vi "Feed Manager.vi"() -> ()   [LabVIEW 2014]
uses:
  _support/Feed Manager States.ctl
  _support/Feed Manager State Data.ctl
  _support/Feed Info.ctl
  _support/UI references.ctl
  <vilib>/Utility/miscctls.llb/LVRowAndColumnTypeDef.ctl
  <vilib>/Utility/miscctls.llb/LVRowAndColumnUnsignedTypeDef.ctl
  <vilib>/National Instruments/NIPM API (Beta)/NIPM_API.lvlib
panel:
  in  "Help Button":bool
  out "Package Attributes":string[][](table)
  in  "Refresh":bool
  in  "Packages in Feed":i32(listbox)=-1
  in  "Unpublish Package":bool
  in  "Publish Package":bool
  in  "Configure Feeds":bool
  in  "Feed":string(combo)="Select a Feed..."
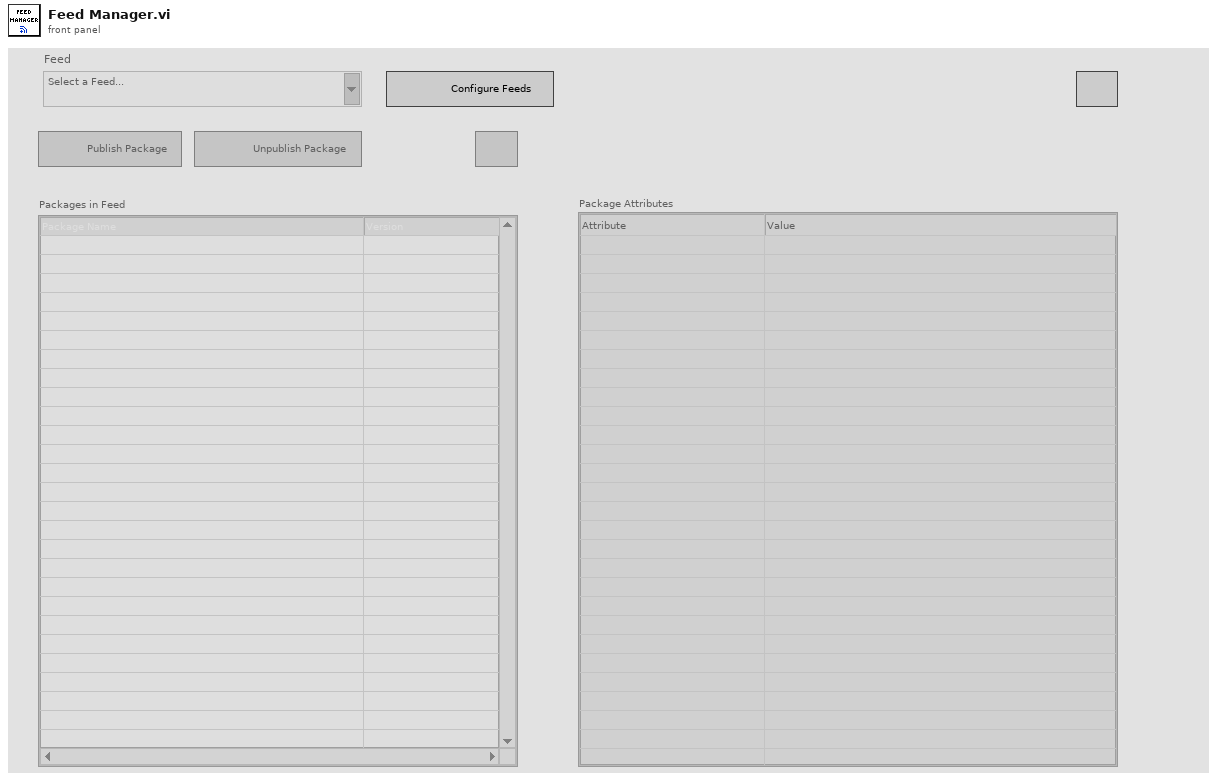
[diagram p1: front panel]
types:
  T1 = typedef "Feed Manager State Data.ctl" = cluster{"Feeds INI Filepath":path, "Current Feed":T2, "Current Row Index":i32, "Managed Feeds":T2[], "Temp Registered Feeds":T2[], "Temp Feed Prefix":string, "Package Relative Filepaths":path[], "UI References":T3}
  T2 = typedef "Feed Info.ctl" = cluster{"Feed Name":string, "Feed Folderpath":string, "Package Destination Folderpath":string}
  T3 = typedef "UI references.ctl" = cluster{"Publish Package":refnum<vi>, "Unpublish Package":refnum<vi>, "Refresh":refnum<vi>, "Packages in Feed":refnum<vi>, "Package Attributes":refnum<vi>}
  T4 = typedef "Feed Manager States.ctl" = enum16{"Initialize", "Wait on Event", "Update Available Feeds", "Configure Feeds", "Update Packages Table", "Update Package Attributes Display", "Publish Package", "Unpublish Package", "Refresh Feed", "Exit"}
  T5 = typedef "LVRowAndColumnTypeDef.ctl" = cluster{"Row":i32, "Column":i32}
  T6 = enum8{"Enabled", "Disabled", "Disabled and Grayed Out"}
  T7 = typedef "LVRowAndColumnUnsignedTypeDef.ctl" = cluster{"Row":u32, "Column":u32}
  T8 = typedef "NIPM_API.lvlib/feed.ctl" = cluster{"Name":string, "URI":string}
  T9 = typedef "NIPM_API.lvlib/package attributes.ctl" = cluster{"Package Name":string, "Display name":string, "Version":string, "Display version":string, "Synopsis":string, "Description":string, "Maintainer":string, "Maintainer email address":string, "Category":string, "Homepage":string, "Release notes":string, "Depends":string[], "Recommends":string[], "Suggests":string[], "Conflicts":string[], "Provides":string[], "Replaces":string[], "Supplements":string[], "Enhances":string[], "Product":bool, "User visible":bool, "Installed size (KB)":u64, "Package filesize (bytes)":u64, "Architecture":string, "Agent":string, "MD5Checksum":string}
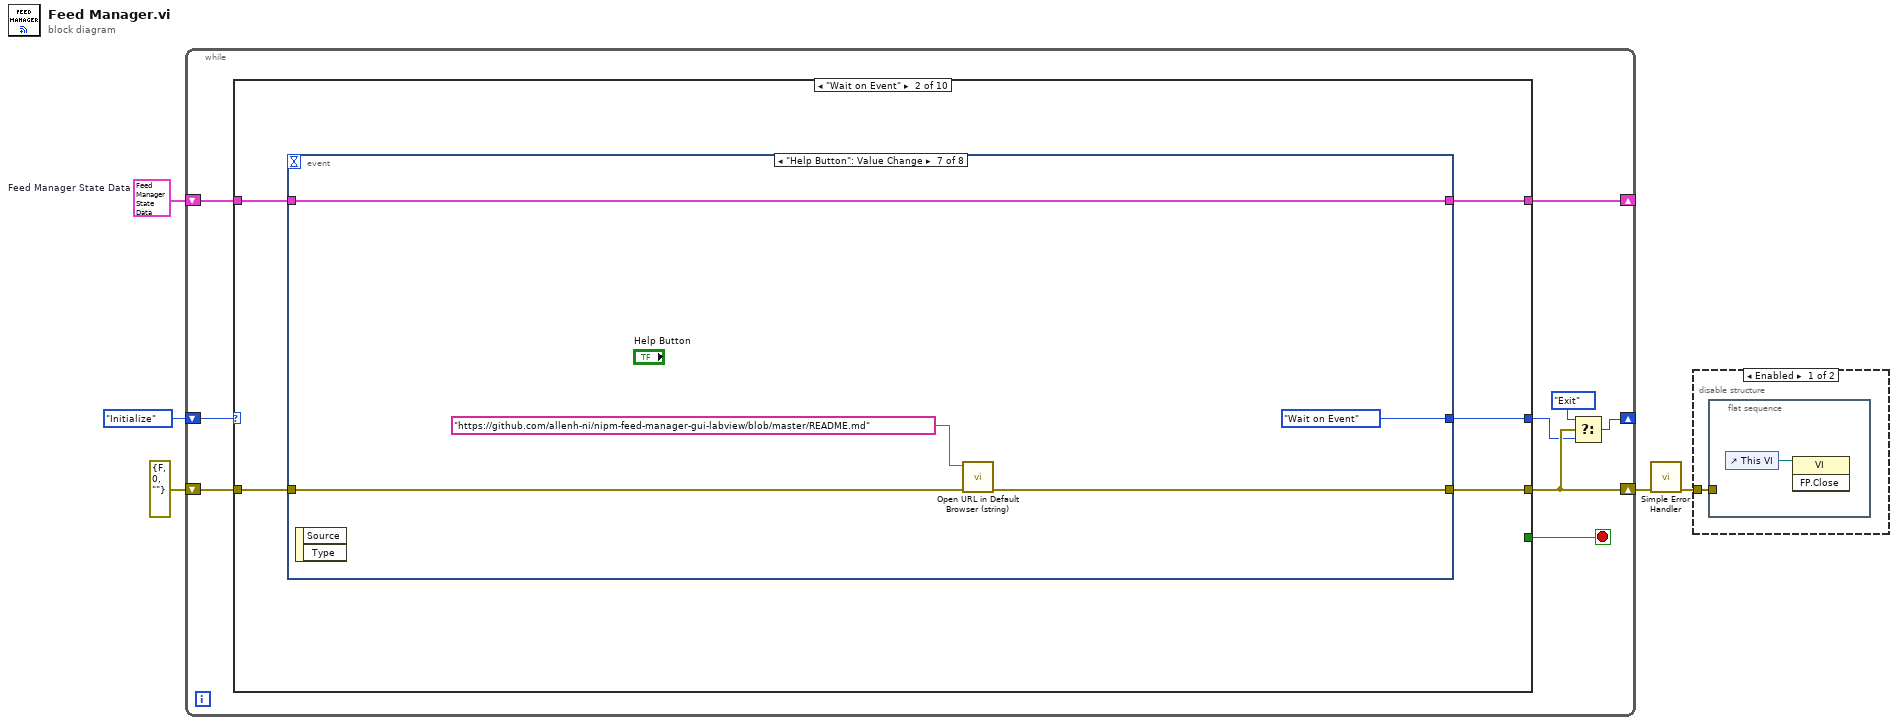
[diagram p0: block diagram]
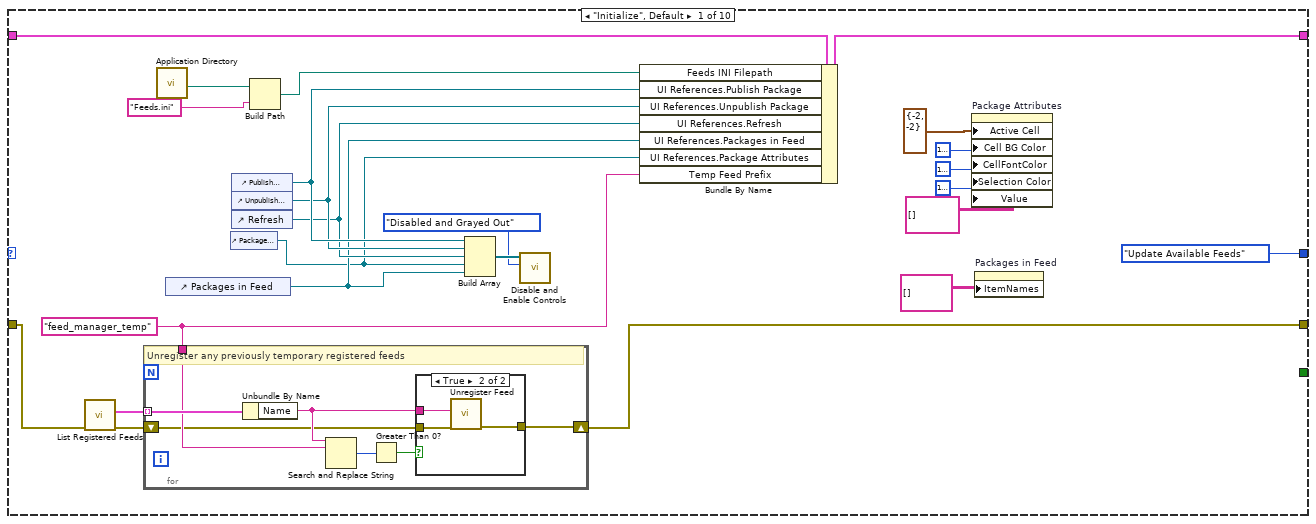
[diagram p3: hidden frame]
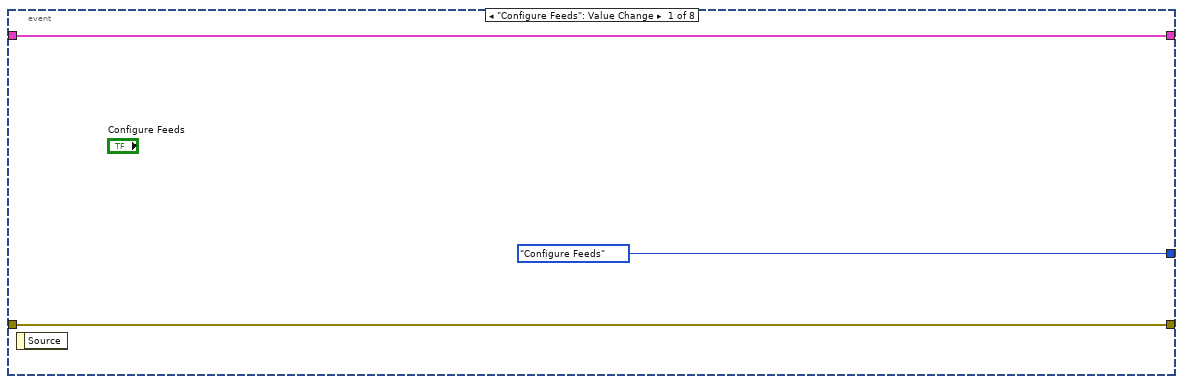
[diagram p5: hidden frame]
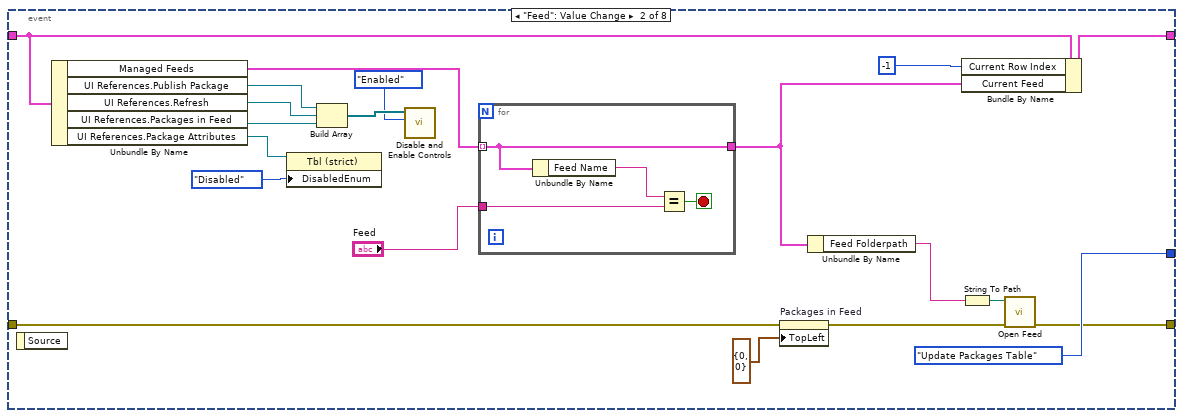
[diagram p6: hidden frame]
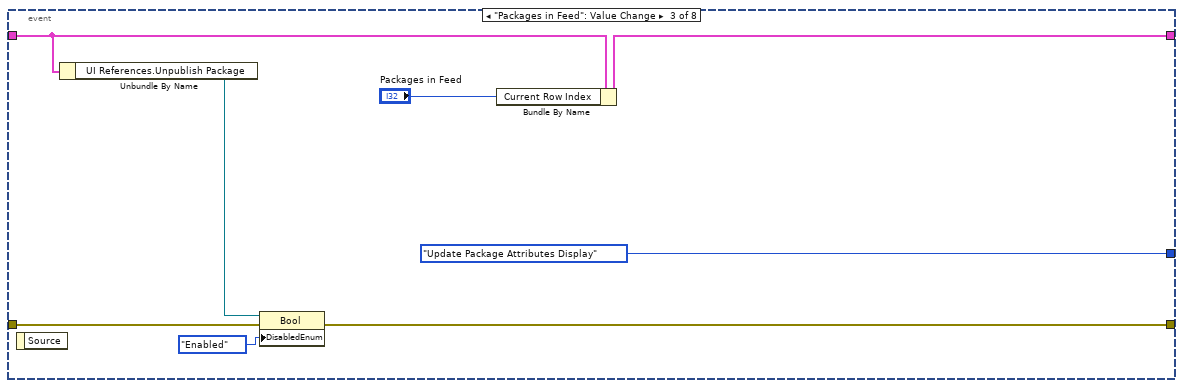
[diagram p7: hidden frame]
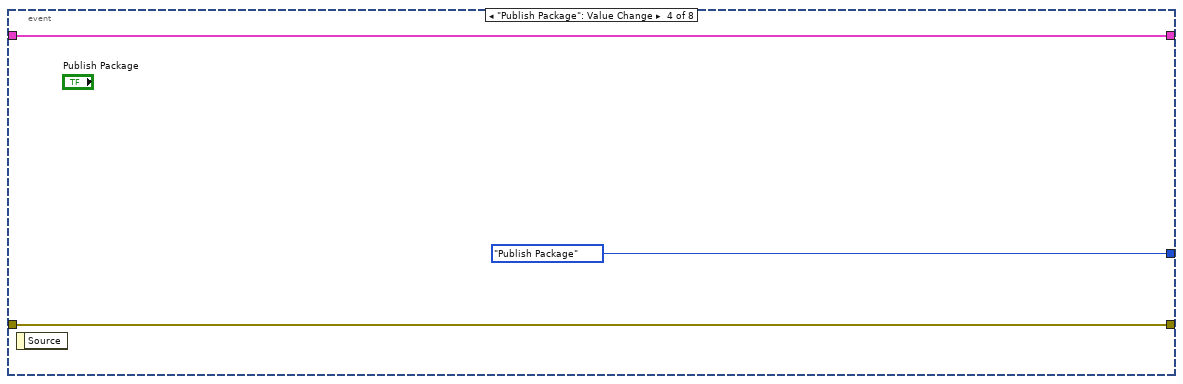
[diagram p8: hidden frame]
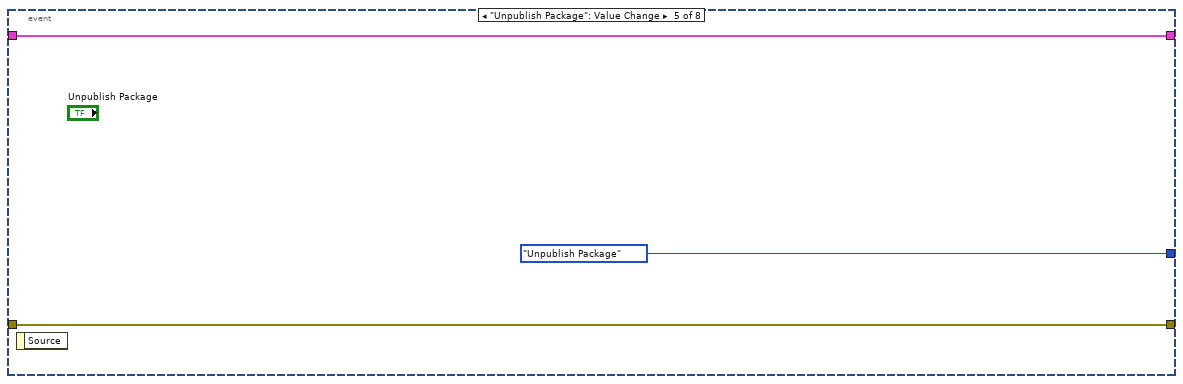
[diagram p9: hidden frame]
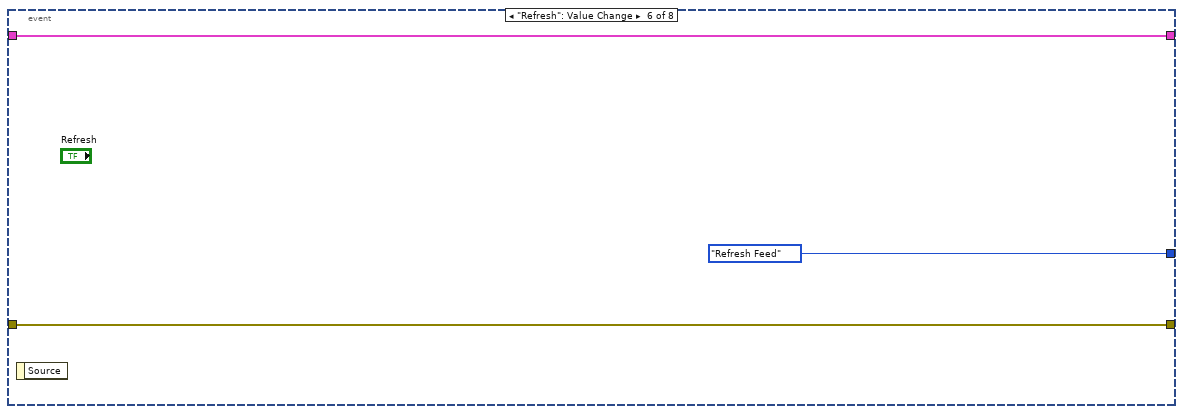
[diagram p10: hidden frame]
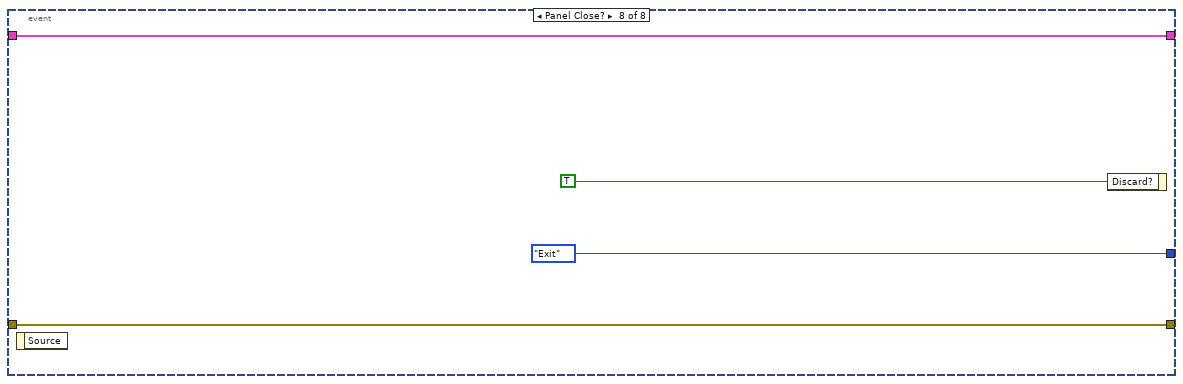
[diagram p11: hidden frame]
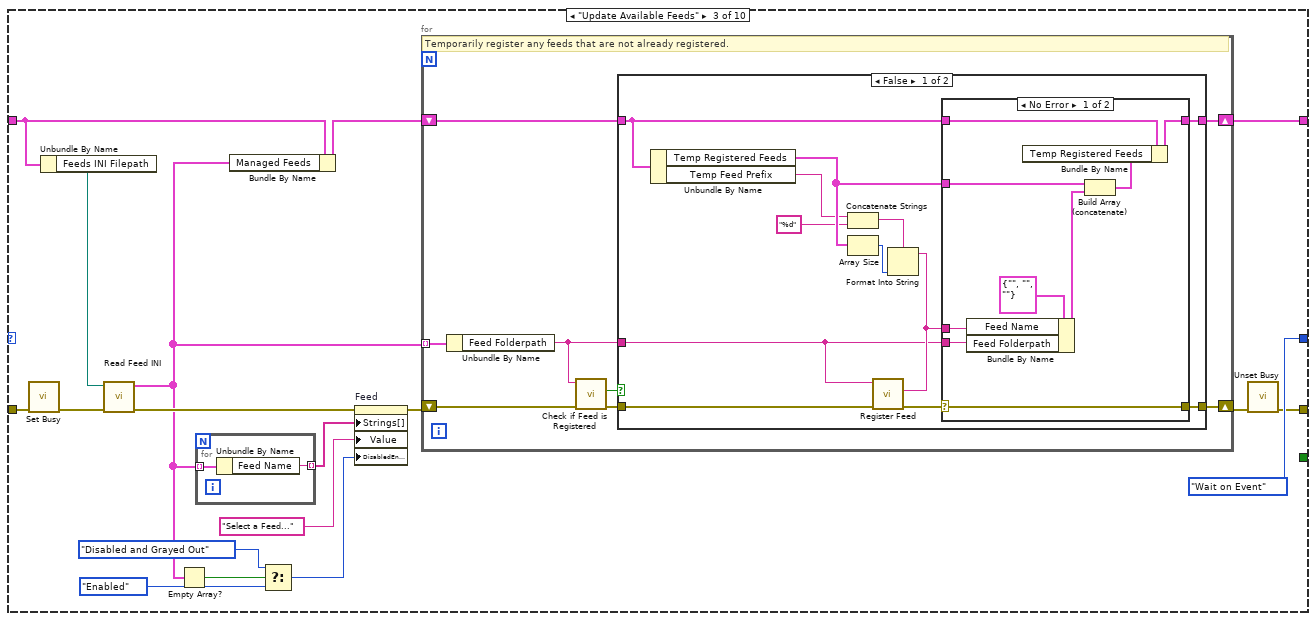
[diagram p12: hidden frame]
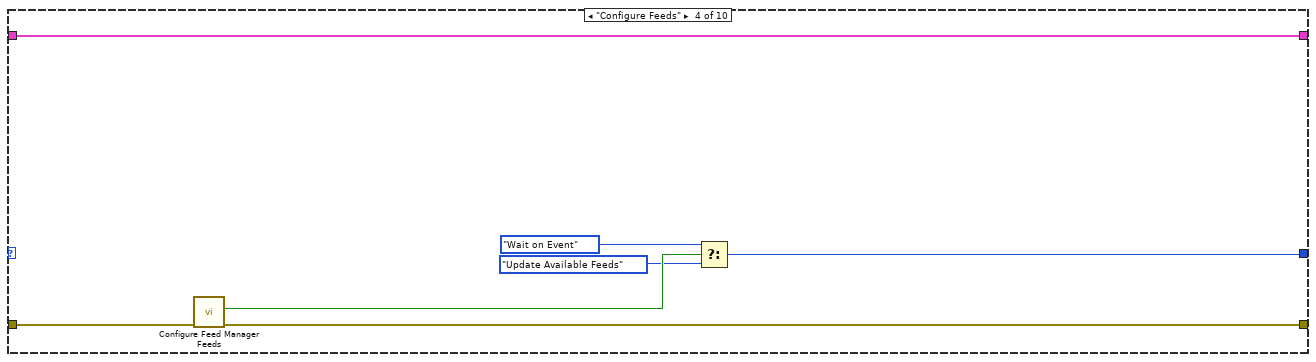
[diagram p15: hidden frame]
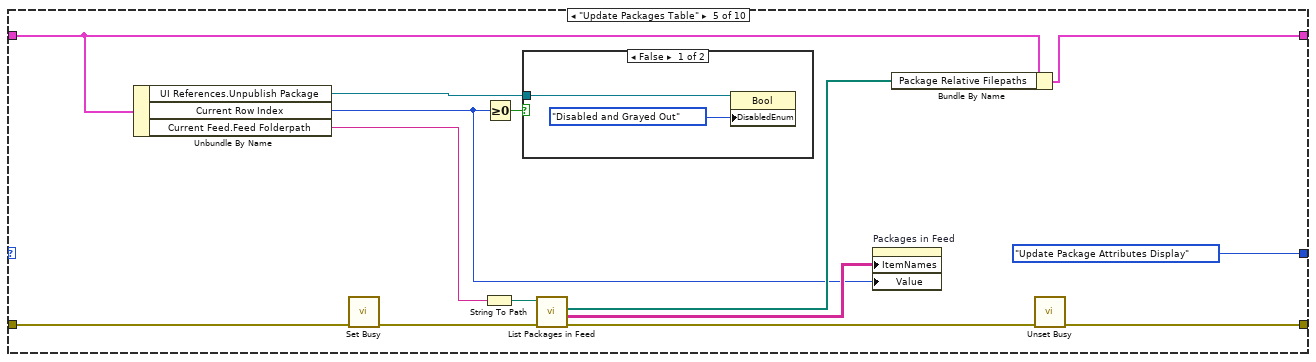
[diagram p16: hidden frame]
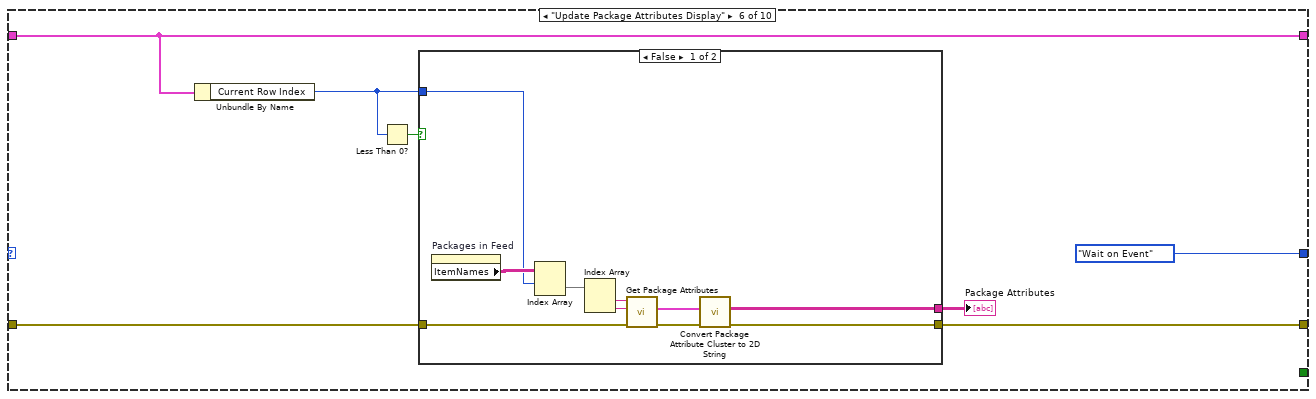
[diagram p18: hidden frame]
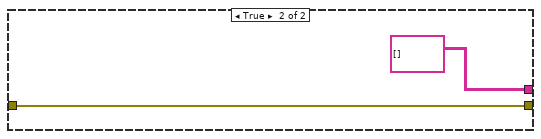
[diagram p19: hidden frame]
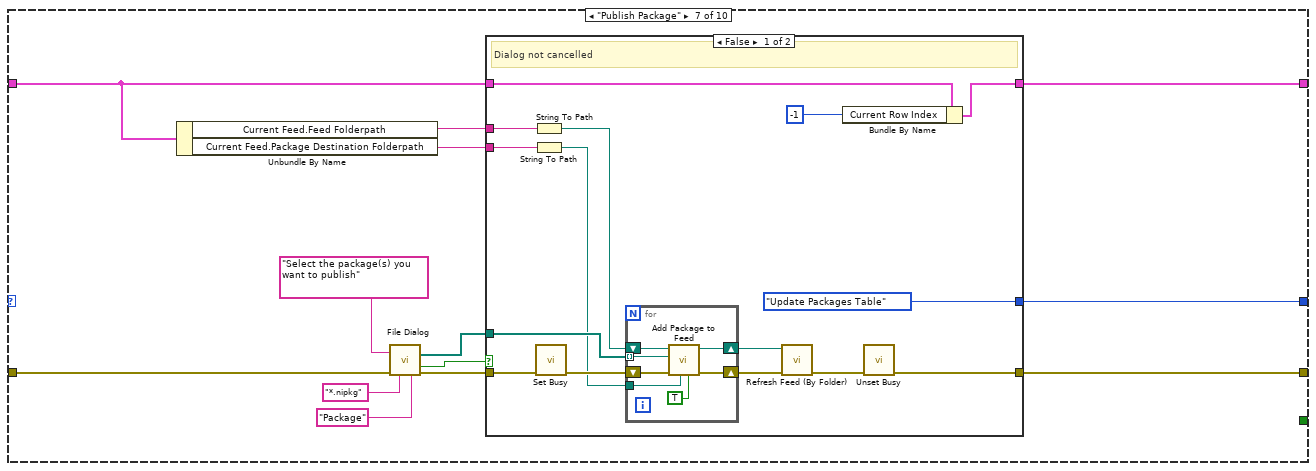
[diagram p20: hidden frame]
diagram:
  w4 = T1 {"Feeds INI Filepath"=path "", "Current Feed"={"Feed Name"="", "Feed Folderpath"="", "Package Destination Folderpath"=""}, "Current Row Index"=-1, "Managed Feeds"=[], "Temp Registered Feeds"=[], "Temp Feed Prefix"="", "Package Relative Filepaths"=[], "UI References"={"Publish Package"=refnum, "Unpublish Package"=refnum, "Refresh"=refnum, "Packages in Feed"=refnum, "Package Attributes"=refnum}}  # Feed Manager State Data
  n1 = while {
    shift-right: [w6] -> _
    shift-left: Feed_Manager_States."Initialize" -> [w14]
    shift-right: [w12] -> _
    shift-left: w4 -> [w13]
    shift-right: [w9] -> w2
    shift-left: errorcluster {"status"=FALSE, "code"=0, "source"=""} ("error in (no error)") -> [w11]
    stop <- w10 stop-if-true
    n2 = case shown="\"Wait on Event\"" w14 {
      tunnel: w13 -> [w38 w53 w118 w167 w179 w188 w206 w256 w273 w286]
      tunnel: [w36 w54 w117 w167 w176 w188 w205 w253 w272 w286] -> w12
      tunnel: [Feed_Manager_States."Update Available Feeds" w50 Feed_Manager_States."Wait on Event" w161 Feed_Manager_States."Update Package Attributes Display" Feed_Manager_States."Wait on Event" w207 Feed_Manager_States."Update Packages Table" Feed_Manager_States."Update Packages Table" Feed_Manager_States."Exit"] -> w8
      tunnel: w11 -> [w16 w52 w125 w163 w178 w190 w210 w257 w276 w289]
      tunnel: [w15 w51 w115 w162 w173 w189 w209 w247 w275 w284] -> w9
      tunnel: [_ _ _ _ _ _ _ _ _ TRUE] -> w10
      frame "Initialize", Default {
        w18 = "feed_manager_temp" ("search string")
        n3 = call <vilib>:"List Registered Feeds.vi"("error in"=w16) -> ("error out"=w17:errorcluster, "registered feeds"=w19:T8[])  [unwired: 9 in]
        n4 = for {
          tunnel: w19 -> [w45] mode=indexing
          tunnel: w18 -> [w44]
          shift-right: [w40] -> w15
          shift-left: w17 -> [w41]
          # "Unregister any previously temporary registered feeds"
          n5 = Unbundle By Name(w45) -> ("Name"=w42:string)
          n6 = Search and Replace String(input string=w42, search string=w44) -> (number of replacements=w43:i32)  [unwired: 6 in, 3 out]
          n7 = Greater Than 0?(x=w43) -> (x > 0?=w39:bool)
          n8 = case shown="True" w39 {
            tunnel: w42 -> [_ w49]
            tunnel: w41 -> [w46 w48]
            tunnel: [w46 w47] -> w40
            frame False {
            }
            frame True {
              n9 = call <vilib>:"Unregister Feed.vi"("error in"=w48, "feed name"=w49) -> ("error out"=w47:errorcluster)  [unwired: 8 in, 1 out]
            }
          }
        }
        n10 = call <vilib>:"Application Directory.vi"() -> ("Application Directory"=w34:path)
        n11 = control-ref of="Packages in Feed"() -> (w22:refnum<vi>)
        n12 = control-ref of="Package Attributes"() -> (w21:refnum<vi>)
        n13 = control-ref of="Publish Package"() -> (w31:refnum<vi>)
        n14 = control-ref of="Unpublish Package"() -> (w30:refnum<vi>)
        n15 = control-ref of="Refresh"() -> (w27:refnum<vi>)
        n16 = Build Path(base path=w34, name or relative path="Feeds.ini") -> (appended path=w33:path)
        n17 = Build Array(w31, w30, w27, w21, w22) -> (w32:refnum<vi>[])
        n18 = call "Disable and Enable Controls.vi"("Disabled"=T6."Disabled and Grayed Out", "Ctrl Refs"=w32) -> ()  [unwired: 10 in]
        n19 = Bundle By Name(cluster=w38, "Feeds INI Filepath"=w33, "UI References.Publish Package"=w31, "UI References.Unpublish Package"=w30, "UI References.Refresh"=w27, "UI References.Packages in Feed"=w22, "UI References.Package Attributes"=w21, "Temp Feed Prefix"=w18) -> (w36:T1)
        n20 = property on="Package Attributes" class="Tbl (strict)"("Active Cell"=T5 {"Row"=-2, "Column"=-2} ("Active Cell:Active Cell"), "Cell BG Color"=u32 16777238, "CellFontColor"=u32 16777222, "Selection Color"=u32 16777224, "Value"=string[][] [] ("Package Attributes")) -> ()  [unwired: 2 in, 2 out]
        n21 = property on="Packages in Feed" class="MCListbox (strict)"("ItemNames"=string[][] [] ("Item Names")) -> ()  [unwired: 2 in, 2 out]
      }
      frame "Wait on Event" {
        n22 = event shown="[6] \"Help Button\": Value Change" {
          selector: _ -> [_ _ _ _ _ _ _ _]
          dyn-events: _ -> [_ _ _ _ _ _ _ _]
          timeout: _ -> [_ _ _ _ _ _ _ _]
          tunnel: [w57 w74 w88 w92 w95 w97 w103 w107] -> w54
          tunnel: w53 -> [w57 w65 w83 w92 w95 w97 w103 w107]
          tunnel: w52 -> [w56 w60 w86 w91 w94 w96 w102 w106]
          tunnel: [w56 w75 w85 w91 w94 w96 w101 w106] -> w51
          tunnel: [Feed_Manager_States."Configure Feeds" Feed_Manager_States."Update Packages Table" Feed_Manager_States."Update Package Attributes Display" Feed_Manager_States."Publish Package" Feed_Manager_States."Unpublish Package" Feed_Manager_States."Refresh Feed" Feed_Manager_States."Wait on Event" Feed_Manager_States."Exit"] -> w50
          event "Configure Feeds": Value Change {
            n23 = event-data() -> ()  [unwired: 1 in, 1 out]
          }
          event "Feed": Value Change {
            n24 = event-data() -> ()  [unwired: 1 in, 1 out]
            n25 = Unbundle By Name(w65) -> ("Managed Feeds"=w64:T2[], "UI References.Publish Package"=w72:refnum<vi>, "UI References.Refresh"=w71:refnum<vi>, "UI References.Packages in Feed"=w69:refnum<vi>, "UI References.Package Attributes"=w67:refnum<vi>)
            n26 = property class="Tbl (strict)"(reference=w67, "DisabledEnum"=T6."Disabled" ("Disabled")) -> ()  [unwired: 1 in, 2 out]
            n27 = Build Array(w72, w71, w69) -> (w70:refnum<vi>[])
            n28 = call "Disable and Enable Controls.vi"("Disabled"=T6."Enabled", "Ctrl Refs"=w70) -> ()  [unwired: 10 in]
            n29 = for {
              tunnel: w64 -> [w78] mode=indexing
              tunnel: "Feed" -> [w80]
              tunnel: [w78] -> w62
              stop <- w79 stop-if-true
              n30 = Unbundle By Name(w78) -> ("Feed Name"=w81:string)
              n31 = Equal?(x=w81, y=w80) -> (x = y?=w79:bool)
            }
            n32 = property on="Packages in Feed" class="MCListbox (strict)"(error in=w60, "TopLeft"=T7 {"Row"=0, "Column"=0} ("Top Left Visible Cell")) -> (error out=w59:errorcluster)  [unwired: 1 in, 1 out]
            n33 = Unbundle By Name(w62) -> ("Feed Folderpath"=w61:string)
            n34 = Bundle By Name(cluster=w65, "Current Row Index"=-1, "Current Feed"=w62) -> (w74:T1)
            n35 = String To Path(string=w61) -> (path=w76:path)
            n36 = call <vilib>:"Open Feed.vi"("error in"=w59, "feed folderpath"=w76) -> ("error out"=w75:errorcluster)  [unwired: 7 in, 2 out]
          }
          event "Packages in Feed": Value Change {
            n37 = event-data() -> ()  [unwired: 1 in, 1 out]
            n38 = Unbundle By Name(w83) -> ("UI References.Unpublish Package"=w84:refnum<vi>)
            n39 = property class="Bool"(reference=w84, error in=w86, "DisabledEnum"=T6."Enabled" ("Disabled")) -> (error out=w85:errorcluster)  [unwired: 1 out]
            n40 = Bundle By Name(cluster=w83, "Current Row Index"="Packages in Feed") -> (w88:T1)
          }
          event "Publish Package": Value Change {
            n41 = event-data() -> ()  [unwired: 1 in, 1 out]
          }
          event "Unpublish Package": Value Change {
            n42 = event-data() -> ()  [unwired: 1 in, 1 out]
          }
          event "Refresh": Value Change {
            n43 = event-data() -> ()  [unwired: 1 in, 1 out]
          }
          event "Help Button": Value Change {
            n44 = event-data() -> ()  [unwired: 1 in, 2 out]
            n45 = call <vilib>:"Open URL in Default Browser (string).vi"("error in (no error)"=w102, "URL"="https://github.com/allenh-ni/nipm-feed-manager-gui-labview/blob/master/README.md") -> ("error out"=w101:errorcluster)  [unwired: 4 in, 1 out]
          }
          event Panel Close? {
            n46 = event-data() -> ()  [unwired: 1 in, 1 out]
            n47 = event-data("Discard?"=TRUE) -> ()  [unwired: 1 in, 1 out]
          }
        }
      }
      frame "Update Available Feeds" {
        n48 = call <vilib>:"Set Busy.vi"("error in (no error)"=w125) -> ("error out"=w116:errorcluster)  [unwired: 9 in, 1 out]
        n49 = Unbundle By Name(w118) -> ("Feeds INI Filepath"=w124:path)
        n50 = call "Read Feed INI.vi"("error in (no error)"=w116, "feed INI filepath"=w124) -> ("error out"=w123:errorcluster, "Feeds"=w112:T2[])  [unwired: 8 in]
        n51 = Empty Array?(array=w112) -> (empty?=w111:bool)
        n52 = for {
          tunnel: w112 -> [w127] mode=indexing
          tunnel: [w126] -> w114 mode=indexing
          n53 = Unbundle By Name(w127) -> ("Feed Name"=w126:string)
        }
        n54 = Bundle By Name(cluster=w118, "Managed Feeds"=w112) -> (w113:T1)
        n55 = Select(t=T6."Disabled and Grayed Out" ("Disabled"), s=w111, f=T6."Enabled" ("Disabled")) -> (s? t:f=w108:T6)
        n56 = property on="Feed" class="CmbBox"(error in=w123, "Strings[]"=w114, "Value"="Select a Feed...", "DisabledEnum"=w108) -> (error out=w122:errorcluster)  [unwired: 1 in, 1 out]
        n57 = for {
          shift-right: [w133] -> w119
          shift-left: w122 -> [w135]
          tunnel: w112 -> [w134] mode=indexing
          shift-right: [w131] -> w117
          shift-left: w113 -> [w132]
          # "Temporarily register any feeds that are not already registered."
          n58 = Unbundle By Name(w134) -> ("Feed Folderpath"=w128:string)
          n59 = call <vilib>:"Check if Feed is Registered.vi"("error in"=w135, "feed URI"=w128) -> ("error out"=w130:errorcluster, "feed URI registered?"=w129:bool)  [unwired: 7 in, 1 out]
          n60 = case shown="False" w129 {
            tunnel: w130 -> [w146 w159]
            tunnel: [w142 w159] -> w133
            tunnel: w132 -> [w145 w160]
            tunnel: [w144 w160] -> w131
            tunnel: w128 -> [w139 _]
            frame False {
              n61 = Unbundle By Name(w145) -> ("Temp Registered Feeds"=w141:T2[], "Temp Feed Prefix"=w138:string)
              n62 = Concatenate Strings(w138, "%d" ("string")) -> (w136:string)
              n63 = Array Size(array=w141) -> (size(s)=w147:i32)
              n64 = Format Into String(format string=w136, w147) -> (resulting string=w140:string)  [unwired: 2 in, 1 out]
              n65 = call <vilib>:"Register Feed.vi"("error in"=w146, "feed name"=w140, "feed URI"=w139) -> ("error out"=w143:errorcluster)  [unwired: 7 in, 1 out]
              n66 = case shown="No Error" w143 {
                selector: w143 -> [w154 w157]
                tunnel: w145 -> [w156 w158]
                tunnel: [w155 w158] -> w144
                tunnel: [w154 w157] -> w142
                tunnel: w141 -> [w153 _]
                tunnel: w140 -> [w150 _]
                tunnel: w139 -> [w149 _]
                frame No Error {
                  n67 = Bundle By Name(cluster=T2 {"Feed Name"="", "Feed Folderpath"="", "Package Destination Folderpath"=""} ("Temp Registered Feeds"), "Feed Name"=w150, "Feed Folderpath"=w149) -> (w148:T2)
                  n68 = Build Array (concatenate)(w153, w148) -> (w152:T2[])
                  n69 = Bundle By Name(cluster=w156, "Temp Registered Feeds"=w152) -> (w155:T1)
                }
                frame Error {
                }
              }
            }
            frame True {
            }
          }
        }
        n70 = call <vilib>:"Unset Busy.vi"("error in (no error)"=w119) -> ("error out"=w115:errorcluster)  [unwired: 10 in]
      }
      frame "Configure Feeds" {
        n71 = call "Configure Feed Manager Feeds.vi"("error in (no error)"=w163) -> ("error out"=w162:errorcluster, "cancelled"=w166:bool)  [unwired: 9 in]
        n72 = Select(t=Feed_Manager_States."Wait on Event", s=w166, f=Feed_Manager_States."Update Available Feeds") -> (s? t:f=w161:T4)
      }
      frame "Update Packages Table" {
        n73 = Unbundle By Name(w179) -> ("UI References.Unpublish Package"=w169:refnum<vi>, "Current Row Index"=w172:i32, "Current Feed.Feed Folderpath"=w171:string)
        n74 = call <vilib>:"Set Busy.vi"("error in (no error)"=w178) -> ("error out"=w174:errorcluster)  [unwired: 9 in, 1 out]
        n75 = String To Path(string=w171) -> (path=w168:path)
        n76 = Greater Or Equal To 0?(x=w172) -> (x >= 0?=w170:bool)
        n77 = case shown="False" w170 {
          tunnel: w169 -> [w182 _]
          frame False {
            n78 = property class="Bool"(reference=w182, "DisabledEnum"=T6."Disabled and Grayed Out" ("Disabled")) -> ()  [unwired: 1 in, 2 out]
          }
          frame True {
          }
        }
        n79 = call <vilib>:"List Packages in Feed.vi"("error in"=w174, "feed folderpath in"=w168) -> ("error out"=w180:errorcluster, "package names and versions"=w181:string[][], "package relative filepaths"=w175:path[])  [unwired: 6 in, 1 out]
        n80 = property on="Packages in Feed" class="MCListbox (strict)"("ItemNames"=w181, "Value"=w172) -> ()  [unwired: 2 in, 2 out]
        n81 = Bundle By Name(cluster=w179, "Package Relative Filepaths"=w175) -> (w176:T1)
        n82 = call <vilib>:"Unset Busy.vi"("error in (no error)"=w180) -> ("error out"=w173:errorcluster)  [unwired: 10 in]
      }
      frame "Update Package Attributes Display" {
        n83 = Unbundle By Name(w188) -> ("Current Row Index"=w186:i32)
        n84 = Less Than 0?(x=w186) -> (x < 0?=w185:bool)
        n85 = case shown="False" w185 {
          tunnel: w190 -> [w196 w202]
          tunnel: [w193 w202] -> w189
          tunnel: w186 -> [w194 _]
          tunnel: [w191 string[][] [] ("package attributes (2D string)")] -> w184
          frame False {
            n86 = property on="Packages in Feed" class="MCListbox (strict)"() -> ("ItemNames"=w197:string[][])  [unwired: 2 in, 2 out]
            n87 = Index Array(array=w197, index (row)=w194) -> (element=w198:string[])  [unwired: 1 in]
            n88 = Index Array(array=w198) -> (element #1=w199:string, element #2=w200:string)  [unwired: 2 in]
            n89 = call <vilib>:"Get Package Attributes.vi"("error in"=w196, "version"=w200, "package name"=w199) -> ("error out"=w195:errorcluster, "package attributes"=w192:T9)  [unwired: 5 in, 2 out]
            n90 = call <vilib>:"Convert Package Attribute Cluster to 2D String.vi"("error in (no error)"=w195, "package attributes (cluster)"=w192) -> ("error out"=w193:errorcluster, "package attributes (2D string)"=w191:string[][])  [unwired: 8 in]
          }
          frame True {
          }
        }
        "Package Attributes" <- w184
      }
      frame "Publish Package" {
        n91 = Unbundle By Name(w206) -> ("Current Feed.Feed Folderpath"=w208:string, "Current Feed.Package Destination Folderpath"=w204:string)
        n92 = call "File Dialog"("prompt"="Select the package(s) you want to publish", "error in"=w210, "pattern (all files)"="*.nipkg", "pattern label"="Package") -> ("selected paths"=w203:path[], "cancelled"=w215:bool, "error out"=w214:errorcluster)  [unwired: 8 in, 1 out]
        n93 = case shown="False" w215 {
          tunnel: w203 -> [w230 _]
          tunnel: w208 -> [w228 _]
          tunnel: w214 -> [w229 w241]
          tunnel: [w224 w239] -> w209
          tunnel: [Feed_Manager_States."Update Packages Table" Feed_Manager_States."Wait on Event"] -> w207
          tunnel: w206 -> [w220 w238]
          tunnel: [w219 w238] -> w205
          tunnel: w204 -> [w218 _]
          frame False {
            # "Dialog not cancelled"
            n94 = String To Path(string=w228) -> (path=w217:path)
            n95 = String To Path(string=w218) -> (path=w216:path)
            n96 = call <vilib>:"Set Busy.vi"("error in (no error)"=w229) -> ("error out"=w225:errorcluster)  [unwired: 9 in, 1 out]
            n97 = for {
              tunnel: w230 -> [w237] mode=indexing
              tunnel: w216 -> [w231]
              shift-right: [w236] -> w226
              shift-left: w225 -> [w235]
              shift-right: [w234] -> w222
              shift-left: w217 -> [w232]
              n98 = call <vilib>:"Add Package to Feed.vi"("create new package destination folderpath if none exists (F)"=TRUE, "package destination folderpath"=w231, "error in"=w235, "package source filepath"=w237, "feed folderpath in"=w232) -> ("error out"=w236:errorcluster, "feed folderpath out"=w234:path)  [unwired: 4 in, 1 out]
            }
            n99 = call <vilib>:"Refresh Feed (By Folder).vi"("error in"=w226, "feed folderpath in"=w222) -> ("error out"=w223:errorcluster)  [unwired: 8 in, 1 out]
            n100 = Bundle By Name(cluster=w220, "Current Row Index"=-1) -> (w219:T1)
            n101 = call <vilib>:"Unset Busy.vi"("error in (no error)"=w223) -> ("error out"=w224:errorcluster)  [unwired: 10 in]
          }
          frame True {
            # "Dialog cancelled"
            n102 = call <vilib>:"Clear Errors.vi"("error in (no error)"=w241, "specific error code to clear (0: all)"=43) -> ("error out"=w239:errorcluster)  [unwired: 4 in, 1 out]
          }
        }
      }
      frame "Unpublish Package" {
        n103 = Unbundle By Name(w256) -> ("Current Feed.Feed Folderpath"=w255:string, "Package Relative Filepaths"=w250:path[], "Current Row Index"=w249:i32)
        n104 = call <vilib>:"Set Busy.vi"("error in (no error)"=w257) -> ("error out"=w245:errorcluster)  [unwired: 9 in, 1 out]
        n105 = Index Array(array=w250, index=w249) -> (element=w258:path)
        n106 = String To Path(string=w255) -> (path=w243:path)
        n107 = Strip Path(path=w258) -> (name=w248:string)  [unwired: 1 out]
        n108 = call <vilib>:"Remove Package from Feed.vi"("error in"=w245, "package filename"=w248, "feed folderpath in"=w243) -> ("error out"=w251:errorcluster, "removed package filepath"=w246:path)  [unwired: 5 in, 2 out]
        n109 = call <vilib>:"Unset Busy.vi"("error in (no error)"=w251) -> ("error out"=w244:errorcluster)  [unwired: 10 in]
        n110 = case shown="No Error" w244 {
          selector: w244 -> [w265 w270]
          tunnel: [w261 w270] -> w247
          tunnel: w246 -> [w259 _]
          frame No Error {
            n111 = Two Button Dialog(message="This package has been removed from the feed.\n\nDo you want to delete the package file also?", 1:"No" ("F button name (\"Cancel\")"), 2:"Yes" ("T button name (\"OK\")")) -> (T button?=w260:bool)
            n112 = case shown="False" w260 {
              tunnel: w265 -> [w266 w269]
              tunnel: [w266 w268] -> w261
              tunnel: w259 -> [_ w267]
              frame False {
              }
              frame True {
                n113 = Delete(path (use dialog)=w267, error in=w269) -> (error out=w268:errorcluster)  [unwired: 3 in, 2 out]
              }
            }
          }
          frame Error {
          }
        }
        n114 = Bundle By Name(cluster=w256, "Current Row Index"=-1) -> (w253:T1)
      }
      frame "Refresh Feed" {
        n115 = Unbundle By Name(w273) -> ("Feeds INI Filepath"=w279:path)
        n116 = call "Read Feed INI.vi"("error in (no error)"=w276, "feed INI filepath"=w279) -> ("error out"=w277:errorcluster, "Feeds"=w278:T2[])  [unwired: 8 in]
        n117 = for {
          tunnel: w278 -> [w283] mode=indexing
          shift-right: [w280] -> w275
          shift-left: w277 -> [w281]
          n118 = Unbundle By Name(w283) -> ("Feed Folderpath"=w282:string)
          n119 = call <vilib>:"Refresh Feed (By URI).vi"("error in (no error)"=w281, "feed URI in"=w282) -> ("error out"=w280:errorcluster)  [unwired: 8 in, 1 out]
        }
        n120 = Bundle By Name(cluster=w273, "Current Row Index"=-1) -> (w272:T1)
      }
      frame "Exit" {
        n121 = Unbundle By Name(w286) -> ("Temp Registered Feeds"=w285:T2[])
        n122 = for {
          shift-right: [w292] -> w284
          shift-left: w289 -> [w293]
          tunnel: w285 -> [w291] mode=indexing
          n123 = Unbundle By Name(w291) -> ("Feed Name"=w290:string)
          n124 = call <vilib>:"Unregister Feed.vi"("error in"=w293, "feed name"=w290) -> ("error out"=w292:errorcluster)  [unwired: 8 in, 1 out]
        }
      }
    }
    n125 = Select(t=Feed_Manager_States."Exit", s=w9, f=w8) -> (s? t:f=w6:T4)
  }
  n126 = call <vilib>:"Simple Error Handler.vi"("error in (no error)"=w2) -> ("error out"=w1:errorcluster)  [unwired: 4 in, 4 out]
  n127 = disable-structure shown="Enabled" {
    disable-tunnel: w1 -> [w294 _]
    frame Enabled {
      n128 = flat-sequence {
        tunnel: w294 -> [_]
        frame #0 {
          n129 = control-ref of="This VI"() -> (w295:refnum<vi>)
          n130 = invoke class="VI" method="FP.Close"(reference=w295) -> ()  [unwired: 2 in, 3 out]
        }
      }
    }
    frame Disabled {
    }
  }
